vi "Advance.vi"(8 "error in (no error)":errorcluster, 11 "TransformTokenizer in":refnum<class "TransformTokenizer.lvclass">) -> (0 "error out":errorcluster, 3 "TransformTokenizer out":refnum<class "TransformTokenizer.lvclass">)   [LabVIEW 2019, in "TransformTokenizer.lvclass"]
uses:
  TransformTokenizer.lvclass
  TransformTokenizer.lvclass/TransformTokenizer.ctl
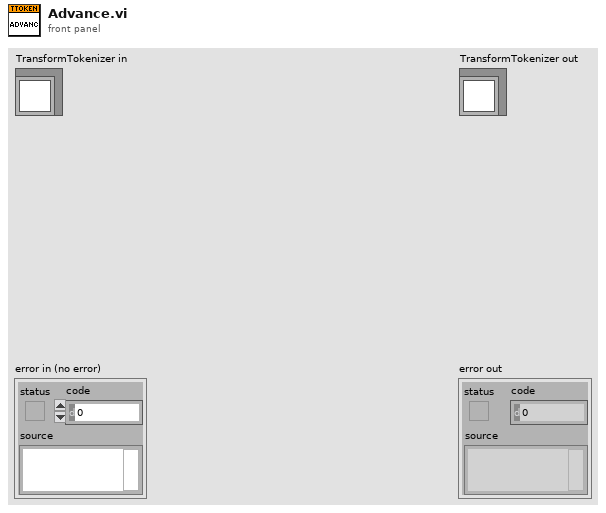
[diagram p1: front panel]
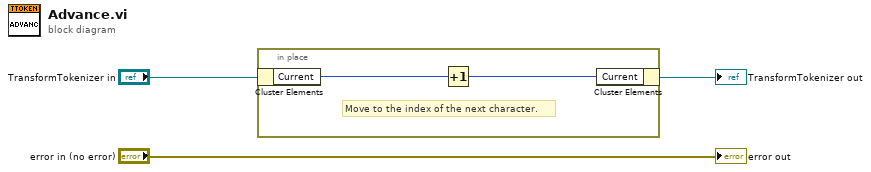
[diagram p0: block diagram]
diagram:
  n1 = in-place {
    # "Move to the index of the next character."
    n2 = in-place-cluster #1("TransformTokenizer in") -> ("Current"=w5:i32)
    n3 = Increment(x=w5) -> (x+1=w4:i32)
    n4 = in-place-cluster #1("Current"=w4) -> (→"TransformTokenizer out":refnum<class "TransformTokenizer.lvclass">)
  }
  "error out" <- "error in (no error)"
